vi "_Read StringList with lvcsm Support.vi"(5 "API Ref":refnum<vi>, 6 "Config Path(\"\" for lvcsm file)":path, 7 "Current Module(\"\" to generate a ID)":string, 8 "error in (no error)":errorcluster, 9 "Force?(F)":bool, 10 "API Name":string="CSMAPI", 11 "CSM Name":string) -> (0 "Error out":errorcluster, 3 "CSMAPI List":string[](array[string]))   [LabVIEW 2017, in "CSM-Helper API with lvcsm Support.lvlib"]
uses:
  CSM-Helper.lvclass
  b7efc127-9b6c-49b9-9e9d-39643bcb625b.vi
  166189b3-b0ee-4f88-bea7-bb947d9812ee.vi
  913c550f-f939-4955-8b9d-1380e6caaad2.vi
  <vilib>/Utility/config.llb/Close Config Data.vi
  <vilib>/Utility/config.llb/Write Key.vi
  <vilib>/Utility/config.llb/Write Key (Double).vi
  <vilib>/Utility/config.llb/Write Key (I32).vi
  <vilib>/Utility/config.llb/Write Key (String).vi
  lvcsmFile/Path to lvcsm String.vi
  <vilib>/Utility/config.llb/Remove Key.vi
  <vilib>/Utility/config.llb/Get Key Names.vi
  Utility/CSM Data Type String.vi
  <vilib>/Utility/config.llb/Write Key (Boolean).vi
  <vilib>/Utility/Data Type/Get Type Information.vi
  <vilib>/Utility/config.llb/Open Config Data.vi
  lvcsmFile/lvcsm File Path.vi
  API/Destroy.vi
  API/Create From VI Reference.vi
  Utility/_openG/Array of VData to VCluster_csm.vi
  <vilib>/Utility/config.llb/Read Key.vi
  <vilib>/Utility/config.llb/Read Key (Double).vi
  <vilib>/Utility/config.llb/Read Key (I32).vi
  lvcsmFile/lvcsm String to Path.vi
  <vilib>/Utility/config.llb/Read Key (String).vi
  <vilib>/Utility/config.llb/Read Key (Boolean).vi
  CSM-Helper API with lvcsm Support.lvlib
  Communicable State Machine.lvlib
  Properties/Read APIs.vi
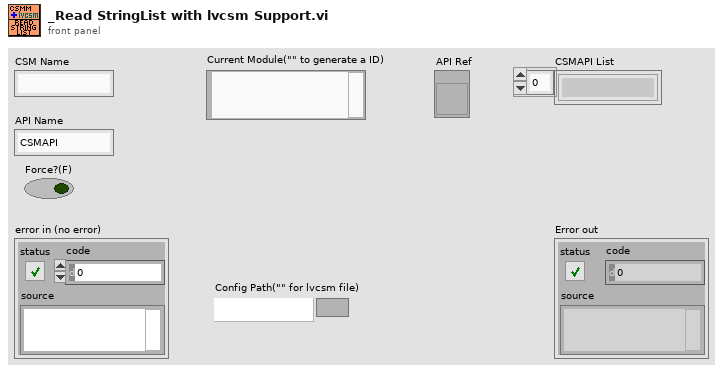
[diagram p1: front panel]
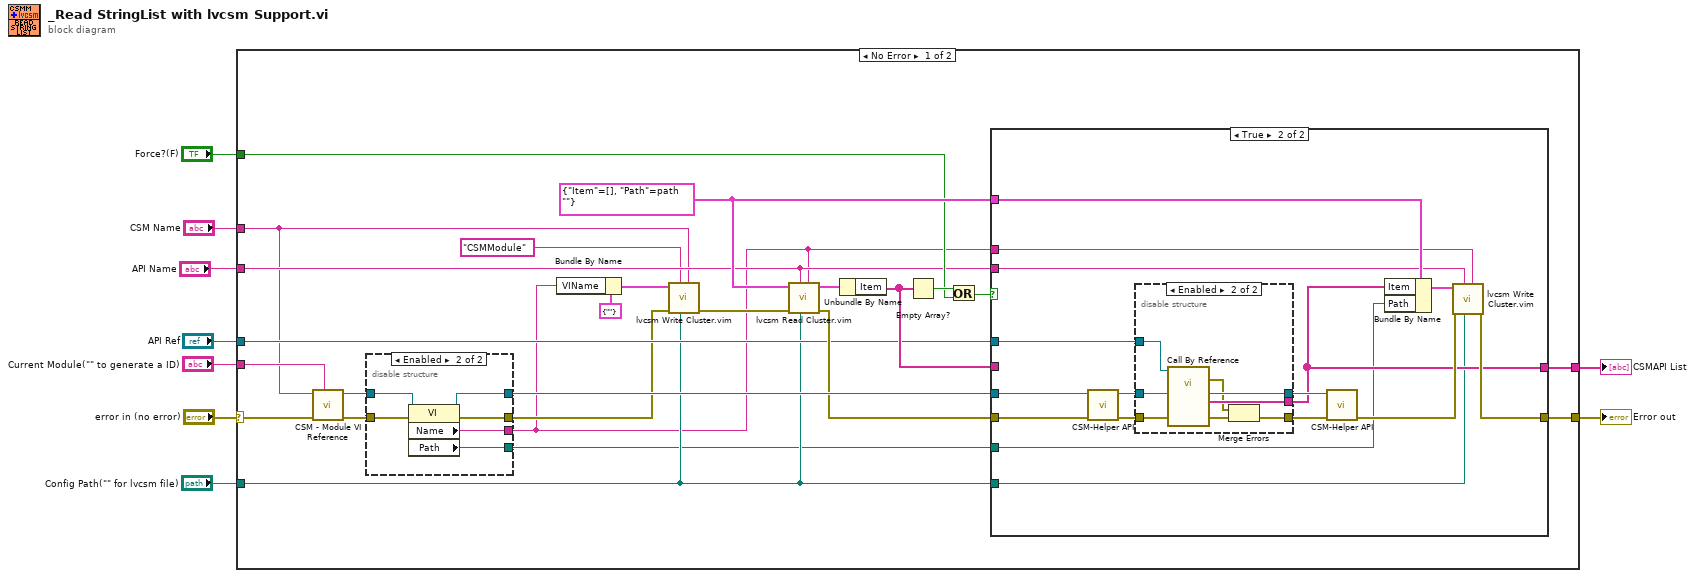
[diagram p0: block diagram]
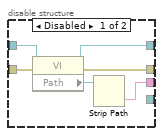
[diagram p2: hidden frame]
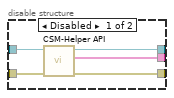
[diagram p4: hidden frame]
diagram:
  n1 = case shown="No Error" "error in (no error)" {
    selector: "error in (no error)" -> [w25 w78]
    tunnel: [w26 w78] -> w9
    tunnel: "CSM Name" -> [w14 _]
    tunnel: "Current Module(\"\" to generate a ID)" -> [w24 _]
    tunnel: [w23 _] -> w5
    tunnel: "Force?(F)" -> [w21 _]
    tunnel: "Config Path(\"\" for lvcsm file)" -> [w17 _]
    tunnel: "API Ref" -> [w20 _]
    tunnel: "API Name" -> [w19 _]
    frame No Error {
      w28 = cluster{"Item":string[], "Path":path} {"Item"=[], "Path"=path ""}
      n2 = call "CSM - Module VI Reference.vi"("Current Module(\"\" to generate a ID)"=w24, "error in (no error)"=w25, "CSM Name"=w14) -> ("error out"=w34:errorcluster, "CSM Module VIRef"=w33:refnum<vi>)  [unwired: 7 in]
      n3 = disable-structure shown="Enabled" {
        disable-tunnel: w34 -> [w40 w46]
        disable-tunnel: w33 -> [w39 w45]
        disable-tunnel: [w38 w44] -> w32
        disable-tunnel: [w36 w43] -> w16
        disable-tunnel: [w35 w42] -> w11
        disable-tunnel: [_ w41] -> w10
        frame Disabled {
          n4 = property class="VI"(reference=w39, error in=w40) -> (reference out=w38:refnum<vi>, error out=w36:errorcluster, "Path"=w37:path)
          n5 = Strip Path(path=w37) -> (name=w35:string)  [unwired: 1 out]
        }
        frame Enabled {
          n6 = property class="VI"(reference=w45, error in=w46) -> (reference out=w44:refnum<vi>, error out=w43:errorcluster, "Name"=w42:string, "Path"=w41:path)
        }
      }
      n7 = Bundle By Name(cluster=cluster{"VIName":string} {"VIName"=""}, "VIName"=w11) -> (w12:cluster{"VIName":string})
      n8 = call "lvcsm Write Cluster.vim"("sub-section(\"\")"=w14, "Config Path"=w17, "Section"="CSMModule", "Error in"=w16, "Configuration"=w12) -> ("Error out"=w18:errorcluster)  [unwired: 6 in]
      n9 = call "lvcsm Read Cluster.vim"("sub-section(\"\")"=w11, "Config Path"=w17, "Section"=w19, "Error in"=w18, "Default Prototype"=w28) -> ("Error out"=w29:errorcluster, "Cluster (dup)"=w31:cluster{"Item":string[], "Path":path})  [unwired: 5 in]
      n10 = Unbundle By Name(w31) -> ("Item"=w27:string[])
      n11 = Empty Array?(array=w27) -> (empty?=w30:bool)
      n12 = Or(x=w30, y=w21) -> (x .or. y?=w22:bool)
      n13 = case shown="True" w22 {
        tunnel: w29 -> [w48 w60]
        tunnel: w32 -> [_ w59]
        tunnel: [w48 w55] -> w26
        tunnel: w28 -> [_ w58]
        tunnel: w19 -> [_ w54]
        tunnel: w11 -> [_ w53]
        tunnel: [w47 w52] -> w23
        tunnel: w27 -> [w47 _]
        tunnel: w17 -> [_ w51]
        tunnel: w20 -> [_ w50]
        tunnel: w10 -> [_ w49]
        frame False {
        }
        frame True {
          n14 = call-poly "CSM-Helper API.vi"("error in (no error)"=w60, "VI"=w59) -> ("error out"=w62:errorcluster, "CSM-Helper.lvclass"=w61:refnum<class "CSM-Helper.lvclass">)  [unwired: 8 in]
          n15 = disable-structure shown="Enabled" {
            disable-tunnel: [w69 w71] -> w64
            disable-tunnel: [w68 w75] -> w63
            disable-tunnel: w62 -> [w67 w74]
            disable-tunnel: w61 -> [w66 w76]
            disable-tunnel: [w65 w72] -> w52
            disable-tunnel: w50 -> [_ w77]
            frame Disabled {
              n16 = call-poly "CSM-Helper API.vi"("error in (no error)"=w67, "CSM-Helper in"=w66) -> ("error out"=w69:errorcluster, "Value"=w65:string[], "CSM-Helper out"=w68:refnum<class "CSM-Helper.lvclass">)  [unwired: 7 in]
            }
            frame Enabled {
              n17 = call-by-ref "?"(reference=w77, "error in (no error)"=w74, "CSM-Helper in"=w76) -> (error out=w70:errorcluster, 0:"error out"=w73:errorcluster, "Value"=w72:string[], "CSM-Helper out"=w75:refnum<class "CSM-Helper.lvclass">)  [unwired: 8 in, 1 out]
              n18 = Merge Errors(w70, w73) -> (w71:errorcluster)
            }
          }
          n19 = call-poly "CSM-Helper API.vi"("error in (no error)"=w64, "CSM-Helper in"=w63) -> ("error out"=w56:errorcluster)  [unwired: 8 in, 1 out]
          n20 = Bundle By Name(cluster=w58, "Item"=w52, "Path"=w49) -> (w57:cluster{"Item":string[], "Path":path})
          n21 = call "lvcsm Write Cluster.vim"("sub-section(\"\")"=w53, "Config Path"=w51, "Section"=w54, "Error in"=w56, "Configuration"=w57) -> ("Error out"=w55:errorcluster)  [unwired: 6 in]
        }
      }
    }
    frame Error {
    }
  }
  "Error out" <- w9
  "CSMAPI List" <- w5
